vi "Define Default Prefix.vi"(8 "error in (no error)":errorcluster, 11 "DI Channel in":refnum<class "DI Channel.lvclass">) -> (0 "error out":errorcluster, 3 "DI Channel out":refnum<class "DI Channel.lvclass">)   [LabVIEW 2017, in "Scan Engine Scripting.lvlib" / "DI Channel.lvclass"]
doc: "Assigns the default prefix to the channel."
uses:
  DI Channel.lvclass
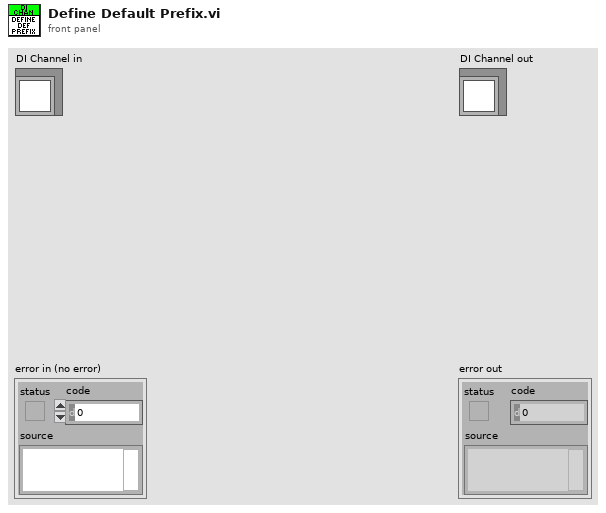
[diagram p1: front panel]
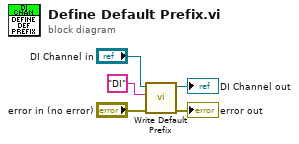
[diagram p0: block diagram]
diagram:
  n1 = call-dynamic "Write Default Prefix.vi"("error in"="error in (no error)", "default prefix"="DI", "channel in"="DI Channel in") -> ("error out"=→"error out":errorcluster, "channel out"=→"DI Channel out":refnum<class "DI Channel.lvclass">)  [unwired: 7 in]
